vi "Create.vi"(10 "col":i32, 11 "row":i32) -> (3 "output cluster":refnum<class "Cell.lvclass">)   [LabVIEW 2021, in "Cell.lvclass"]
uses:
  Cell.lvclass
  TypeDefs/Cell Status.ctl
  Cell.lvclass/Cell.ctl
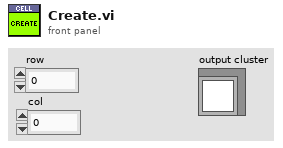
[diagram p1: front panel]
types:
  T1 = typedef "Cell.lvclass/Cell Status.ctl" = enum16{"default", "selected", "completed"}
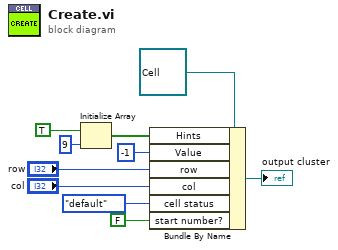
[diagram p0: block diagram]
diagram:
  n1 = Initialize Array(TRUE, 9 ("dimension size")) -> (w2:bool[])
  n2 = Bundle By Name(cluster=refnum<class "Cell.lvclass"> refnum ("Cell.lvclass"), "Hints"=w2, "Value"=i8 -1, "row"="row", "col"="col", "cell status"=Cell_Status."default", "start number?"=FALSE ("number known?")) -> (→"output cluster":refnum<class "Cell.lvclass">)
